vi "Do.vi"(8 "error in (no error)":errorcluster, 10 "Actor in":refnum<class "Actor.lvclass">, 11 "Remove Cashier Msg":refnum<class "Remove Cashier Msg.lvclass">) -> (0 "error out":errorcluster, 2 "Actor out":refnum<class "Actor.lvclass">)   [LabVIEW 2023, in "Coffee Shop.lvlib" / "Remove Cashier Msg.lvclass"]
doc: "This VI delivers the message to the actor by calling the appropriate method(s) on the actor."
uses:
  Remove Cashier Msg.lvclass
  <vilib>/ActorFramework/Actor/Actor.lvclass
  Coffee Shop/Coffee Shop.lvclass
  c:/dev/_r/4/eng/lv-core/lvpostprocessingd/lv_mc_x86_64/dist_i386/vi.lib/ActorFramework/Actor/Actor.lvclass
  Remove Cashier Msg.lvclass/Remove Cashier Msg.ctl
  Coffee Shop/Entity Types.ctl
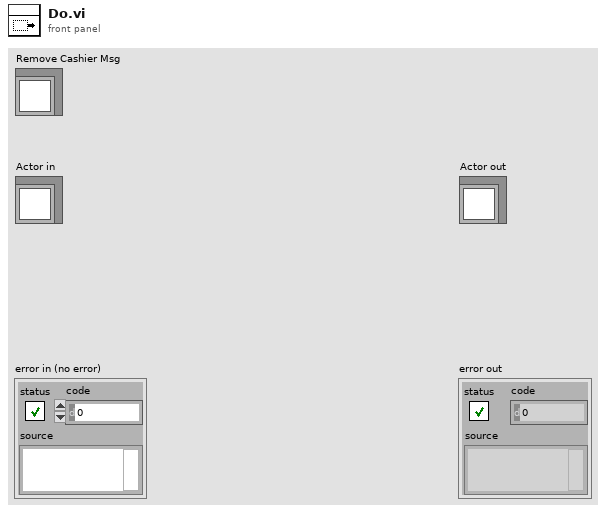
[diagram p1: front panel]
types:
  T1 = typedef "Coffee Shop.lvlib/Coffee Shop.lvclass/Entity Types.ctl" = enum16{"Customer", "Cashier", "Barista"}
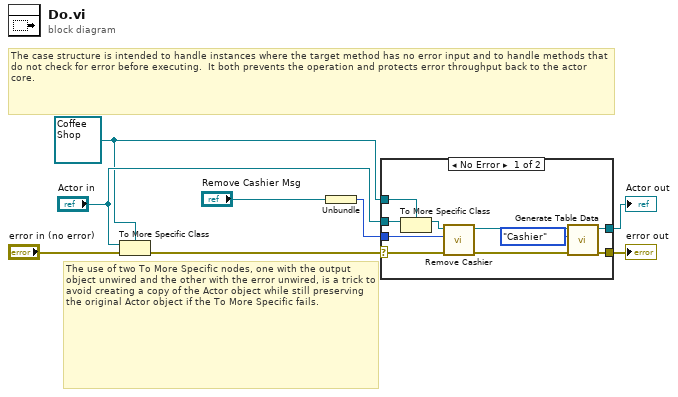
[diagram p0: block diagram]
diagram:
  w2 = refnum<class "Coffee Shop.lvclass"> refnum ("Actor in")
  # "The use of two To More Specific nodes, one with the output object unwired and the other with the error unwired, is a trick to avoid creating a copy of the Actor object while still preserving the original Actor object if the To More Specific fails."
  # "The case structure is intended to handle instances where the target method has no error input and to handle methods that do not check for error before executing.  It both prevents the operation and protects error throughput back to the actor core."
  n1 = To More Specific Class(target class=w2, reference="Actor in", error in="error in (no error)") -> (error out=w6:errorcluster)  [unwired: 1 out]
  n2 = Unbundle("Remove Cashier Msg") -> (w1:i32)
  n3 = case shown="No Error" w6 {
    selector: w6 -> [w18 w20]
    tunnel: [w13 w20] -> w5
    tunnel: [w12 w19] -> w4
    tunnel: "Actor in" -> [w17 w19]
    tunnel: w2 -> [w16 _]
    tunnel: w1 -> [w14 _]
    frame No Error {
      n4 = To More Specific Class(target class=w16, reference=w17) -> (specific class reference=w15:refnum<class "Coffee Shop.lvclass">)  [unwired: 1 in, 1 out]
      n5 = call-dynamic "Remove Cashier.vi"("error in (no error)"=w18, "Cashier Index"=w14, "Coffee Shop in"=w15) -> ("error out"=w10:errorcluster, "Coffee Shop out"=w11:refnum<class "Coffee Shop.lvclass">)  [unwired: 7 in]
      n6 = call-dynamic "Generate Table Data.vi"("error in (no error)"=w10, "Entity Type"=Entity_Types."Cashier", "Coffee Shop in"=w11) -> ("error out"=w13:errorcluster, "Coffee Shop out"=w12:refnum<class "Coffee Shop.lvclass">)  [unwired: 7 in]
    }
    frame Error {
      # "If type check fails, pass the original object out again."
    }
  }
  "error out" <- w5
  "Actor out" <- w4
